vi "Test Lockin Engine.vi"(8 "error in (no error)":errorcluster, 11 "Lockin.DAQ":refnum<class "Instrument.DAQ.lvclass">) -> (0 "error out":errorcluster, 3 "Lockin.DAQ":refnum<class "Instrument.DAQ.lvclass">)   [LabVIEW 2019, in "Instrument.Lockin.lvlib" / "Instrument.DAQ.lvclass"]
uses:
  Instrument.DAQ.lvclass
  DAQmx/DAQmx.lvclass
  <vilib>/Analysis/NI_AALBase.lvlib
  <vilib>/Analysis/baseanly.llb/Mean (DBL).vi
  C:/Program Files/National Instruments/LabVIEW 2019/vi.lib/JKI/JKI SMO/SMO/SMO.lvclass
  Typedefs/AO.Channel.Function--Enum.ctl
  Typedefs/AO.Channel--Cluster--Array.ctl
  Typedefs/DAQ.Sampling.Sampling--Cluster.ctl
  Typedefs/AO.Channel--Cluster.ctl
  Typedefs/REF.Channel--Cluster.ctl
  Typedefs/REF.Channel--Cluster--Array.ctl
  Typedefs/AI.Channel--Cluster.ctl
  Typedefs/AI.Channel--Cluster--Array.ctl
panel:
  in  "Configuration.AI Channels":T1=[{"Enable?"=TRUE, "Channel"=1, "References"=[1], "reference index"=0}] {"reference index" min=1; "References" items=["", "1", "2", "3", "4", "5", "6", "7", "8", "9"]; "Channel" min=1}
  in  "Configuration.Channels: REF":T3=[{"Enable?"=TRUE, "Channel"=1, "Frequency"=13.0, "Phase"=0.0, "TC"=0.1, "Roll-Off"=2}] {"Roll-Off" min=1 max=4; "TC" min=1e-06 max=100.0 format="%#_3p"; "Phase" format="%#_3p"; "Frequency" min=1e-06 max=102400.0 format="%#_6p"; "Channel" min=1}
  out "refresh rate (Hz)":dbl=13.0
  out "Waveform Graph":dbl[][](graph)=[[0.007605197078202029, 0.03790640341016081, 0.068814310341492]]
  in  "buffer size (samples)":i32=100
  in  "intervals":i32=10
  out "Histogram Graph":T5(graph)
  in  "sampling":T6={"Fs"=204789.0, "#s"=15753} {"Fs" format="%#_13g"}
  in  "Type":enum16{"X", "Y", "R", "Theta", "Mean"}(ring)
  in  "stop":bool
  out "Average time (ms)":dbl=2.3333333333333335
  out "Waveform Chart 2":dbl(graph)
  out "Waveform Chart":dbl[][](graph)=[[0.068814310341492]]
  in  "AO Channels":T7=[{"Enable?"=FALSE, "Channel"=1, "Amplitude"=0.1, "Offset"=0.0, "Frequency"=13.0, "Phase"=0.0, "Function"=enum."sine", "Sweeping?"=FALSE, "Limit AC"=FALSE, "Limit DC?"=FALSE, "Duty Cycle"=FALSE}] {"Phase" format="%#_3g"; "Frequency" min=0.0001 max=200000.0 format="%#_6p"; "Offset" format="%#_6p"; "Amplitude" min=0.0 max=10.0 format="%#_6p"}
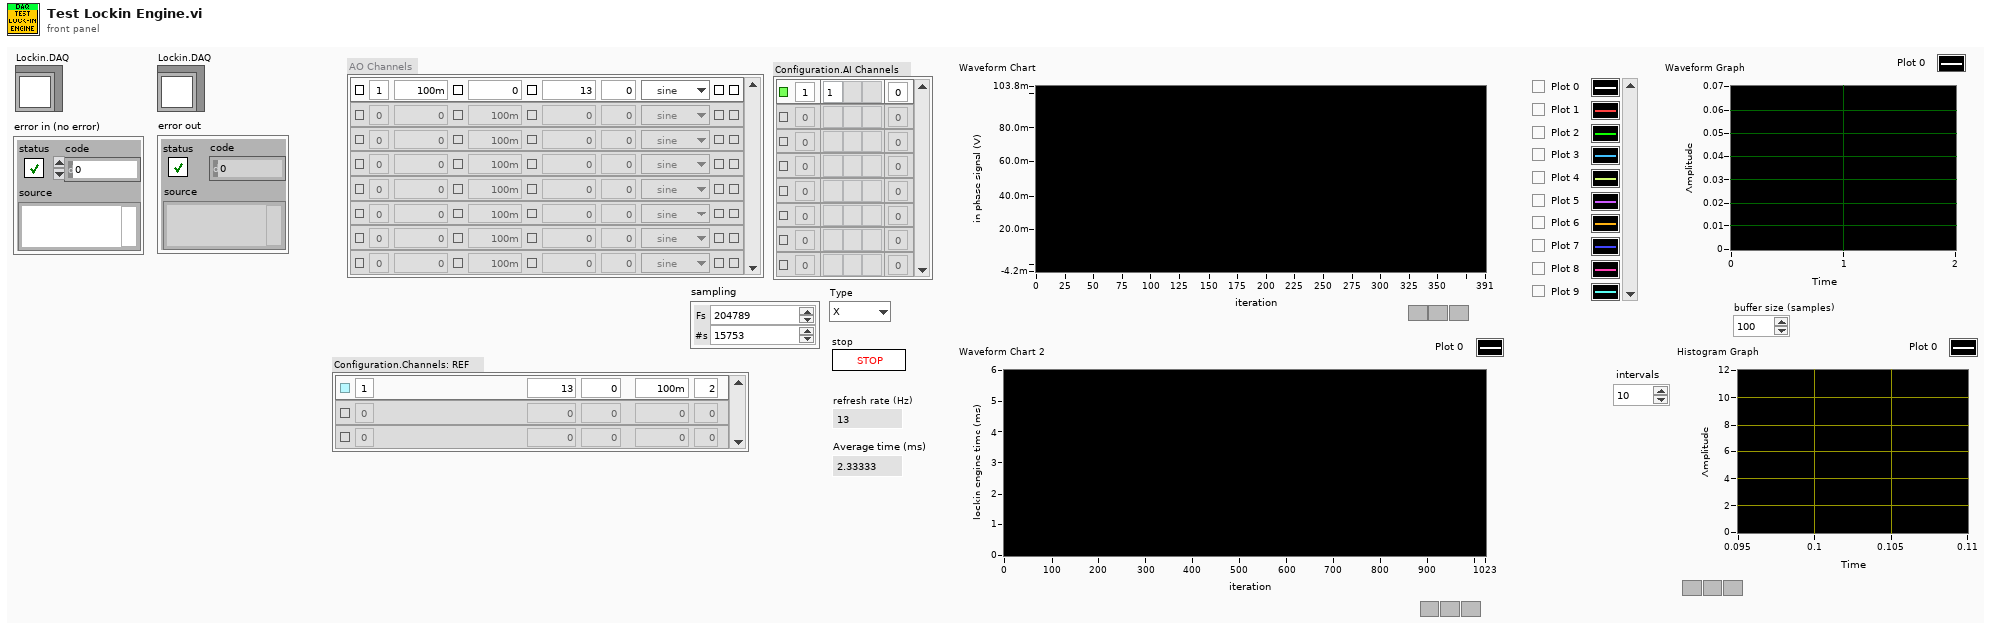
[diagram p1: front panel]
types:
  T1 = typedef "Instrument.Lockin.lvlib/Instrument.DAQ.lvclass/AI.Channel--Cluster--Array.ctl" = T2[]
  T2 = typedef "Instrument.Lockin.lvlib/Instrument.DAQ.lvclass/AI.Channel--Cluster.ctl" = cluster{"Enable?":bool, "Channel":i32, "References":u16[], "reference index":i32}
  T3 = typedef "Instrument.Lockin.lvlib/Instrument.DAQ.lvclass/REF.Channel--Cluster--Array.ctl" = T4[]
  T4 = typedef "Instrument.Lockin.lvlib/Instrument.DAQ.lvclass/REF.Channel--Cluster.ctl" = cluster{"Enable?":bool, "Channel":i32, "Frequency":dbl, "Phase":dbl, "TC":dbl, "Roll-Off":i32}
  T5 = cluster{"X Values":dbl[], "Histogram: h(x)":i32[]}[]
  T6 = typedef "Instrument.Lockin.lvlib/Instrument.DAQ.lvclass/DAQ.Sampling.Sampling--Cluster.ctl" = cluster{"Fs":dbl, "#s":i32}
  T7 = typedef "Instrument.Lockin.lvlib/Instrument.DAQ.lvclass/AO.Channel--Cluster--Array.ctl" = T8[]
  T8 = typedef "Instrument.Lockin.lvlib/Instrument.DAQ.lvclass/AO.Channel--Cluster.ctl" = cluster{"Enable?":bool, "Channel":i32, "Amplitude":dbl, "Offset":dbl, "Frequency":dbl, "Phase":dbl, "Function":T9, "Sweeping?":bool, "Limit AC":bool, "Limit DC?":bool, "Duty Cycle":bool}
  T9 = typedef "Instrument.Lockin.lvlib/Instrument.DAQ.lvclass/AO.Channel.Function--Enum.ctl" = enum16{"sine", "square", "triangle", "saw"}
  T10 = typedef "Instrument.Lockin.lvlib/Instrument.DAQ.lvclass/Results--Cluster.ctl" = cluster{"Time Stamp":timestamp, "Results (Dictionary)":cluster{"key":string, "value":dbl[]}[]}
  T11 = cluster{"X Values":dbl[], "Histogram: h(x)":i32[]}
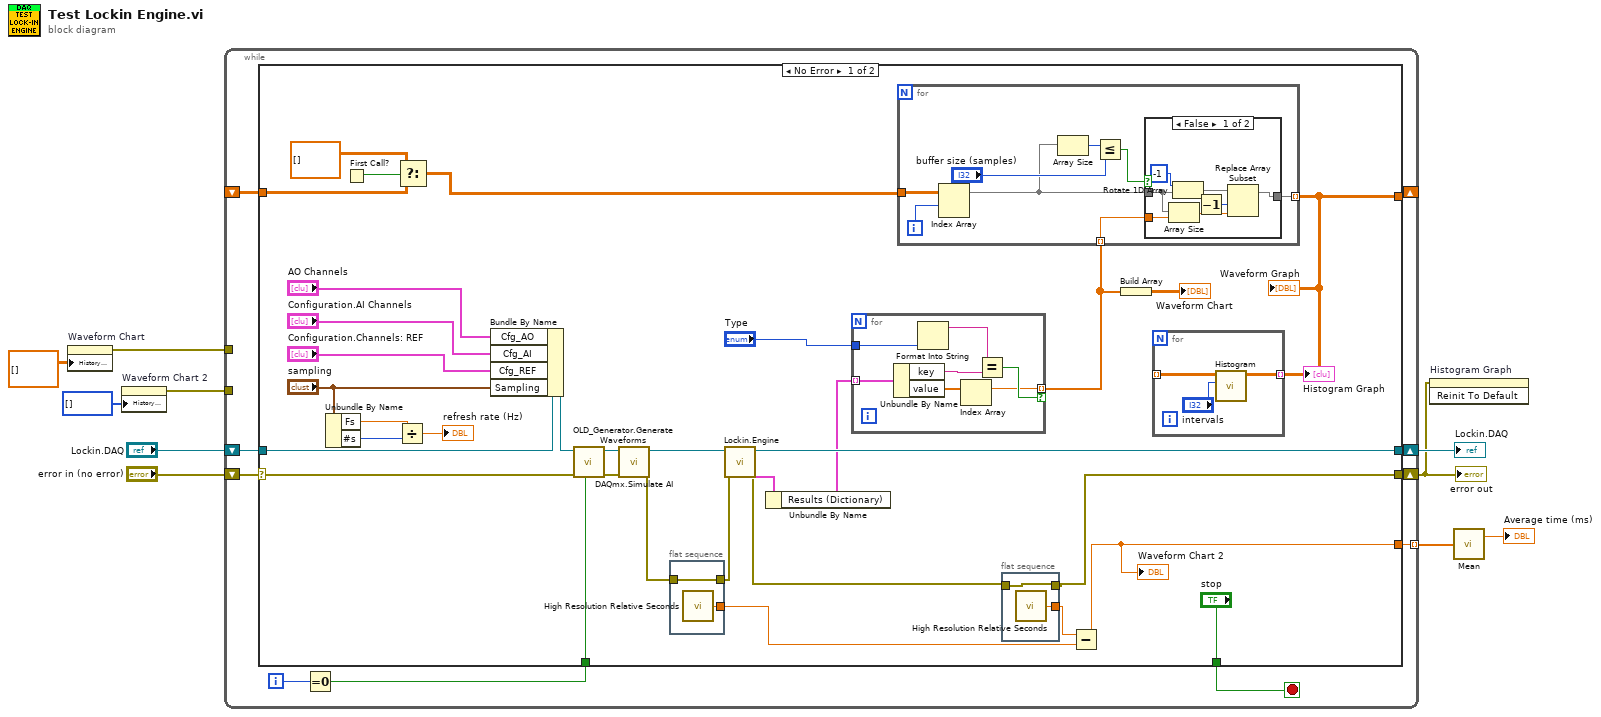
[diagram p0: block diagram]
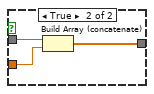
[diagram p2: hidden frame]
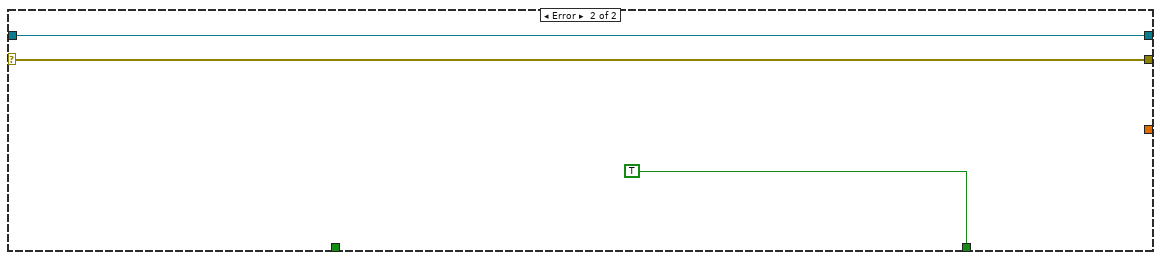
[diagram p3: hidden frame]
diagram:
  n1 = property on="Waveform Chart" class="WFChart (strict)"("History Data"=dbl[][] []) -> (error out=w3:errorcluster)  [unwired: 2 in, 1 out]
  n2 = property on="Waveform Chart 2" class="WFChart (strict)"("History Data"=u32[] []) -> (error out=w4:errorcluster)  [unwired: 2 in, 1 out]
  n3 = while {
    shift-right: [w19] -> w1
    shift-left: "error in (no error)" -> [w20]
    shift-right: [w17] -> w8
    shift-left: "Lockin.DAQ" -> [w18]
    tunnel: [w16] -> w5 mode=indexing
    tunnel: w4 -> [_]
    tunnel: w3 -> [_]
    shift-right: [w12] -> _
    shift-left: _ -> [w11]
    i -> [w14]
    stop <- w13 stop-if-true
    n4 = Equal To 0?(x=w14) -> (x = 0?=w15:bool)
    n5 = case shown="No Error" w20 {
      selector: w20 -> [w53 w89]
      tunnel: [w21 w89] -> w19
      tunnel: [w51 w88] -> w17
      tunnel: w18 -> [w32 w88]
      tunnel: [w48 _] -> w16
      tunnel: w15 -> [w46 _]
      tunnel: ["stop" TRUE ("stop")] -> w13
      tunnel: [w44 _] -> w12
      tunnel: w11 -> [w39 _]
      frame No Error {
        n6 = Unbundle By Name("sampling") -> ("Fs"=w38:dbl, "#s"=w37:i32)
        n7 = First Call?() -> (First Call?: T/F=w41:bool)
        n8 = Divide(x=w38, y=w37) -> (x/y=→"refresh rate (Hz)":dbl)
        n9 = Select(t=dbl[][] [], s=w41, f=w39) -> (s? t:f=w40:dbl[][])
        n10 = Bundle By Name(cluster=w32, "Cfg_AO"="AO Channels", "Cfg_AI"="Configuration.AI Channels", "Cfg_REF"="Configuration.Channels: REF", "Sampling"="sampling") -> (w34:refnum<class "Instrument.DAQ.lvclass">)
        n11 = call "OLD_Generator.Generate Waveforms.vi"("reset phase?"=w46, "error in (no error)"=w53, "Instrument.DAQ"=w34) -> ("error out"=w30:errorcluster, "Instrument.DAQ"=w54:refnum<class "Instrument.DAQ.lvclass">)  [unwired: 6 in, 1 out]
        n12 = call "DAQmx.Simulate AI.vi"("error in (no error)"=w30, "DAQmx in"=w54) -> ("error out"=w23:errorcluster, "DAQmx out"=w52:refnum<class "DAQmx.lvclass">)  [unwired: 6 in, 2 out]
        n13 = flat-sequence {
          tunnel: [w58] -> w28
          tunnel: [w57] -> w24
          tunnel: w23 -> [w57]
          frame #0 {
            n14 = call <vilib>:"High Resolution Relative Seconds.vi"() -> ("relative seconds"=w58:dbl)
          }
        }
        n15 = call "Lockin.Engine.vi"("error in (no error)"=w24, "Instrument.DAQ"=w52) -> ("error out"=w22:errorcluster, "Results (X,Y,R,Theta,Mean)"=w50:T10, "Instrument.DAQ out"=w51:refnum<class "Instrument.DAQ.lvclass">)  [unwired: 5 in, 2 out]
        n16 = Unbundle By Name(w50) -> ("Results (Dictionary)"=w27:cluster{"key":string, "value":dbl[]}[])
        n17 = for {
          tunnel: w27 -> [w65] mode=indexing
          tunnel: "Type" -> [w64]
          tunnel: [w59] -> w25 mode=indexing if=w60
          n18 = Unbundle By Name(w65) -> ("key"=w62:string, "value"=w61:dbl[])
          n19 = Format Into String(w64) -> (resulting string=w63:string)  [unwired: 3 in, 1 out]
          n20 = Index Array(array=w61) -> (element=w59:dbl)  [unwired: 1 in]
          n21 = Equal?(x=w63, y=w62) -> (x = y?=w60:bool)
        }
        n22 = for {
          tunnel: w40 -> [w76]
          tunnel: [w72] -> w44 mode=indexing
          tunnel: w25 -> [w71] mode=indexing
          i -> [w69]
          n23 = Index Array(array=w76, index (row)=w69) -> (element=w70:dbl[])  [unwired: 1 in]
          n24 = Array Size(array=w70) -> (size(s)=w75:i32)
          n25 = Less Or Equal?(x=w75, y="buffer size (samples)") -> (x <= y?=w73:bool)
          n26 = case shown="False" w73 {
            tunnel: [w78 w86] -> w72
            tunnel: w71 -> [w81 w84]
            tunnel: w70 -> [w80 w85]
            frame False {
              n27 = Array Size(array=w80) -> (size(s)=w79:i32)
              n28 = Rotate 1D Array(1:w80, 2:-1 ("n")) -> (0:w82:dbl[])
              n29 = Decrement(x=w79) -> (x-1=w77:i32)
              n30 = Replace Array Subset(array=w82, new element=w81, index=w77) -> (w78:dbl[])
            }
            frame True {
              n31 = Build Array (concatenate)(w85, w84) -> (w86:dbl[])
            }
          }
        }
        "Waveform Graph" <- w44
        n32 = flat-sequence {
          tunnel: [w56] -> w49
          tunnel: [w55] -> w21
          tunnel: w22 -> [w55]
          frame #0 {
            n33 = call <vilib>:"High Resolution Relative Seconds.vi"() -> ("relative seconds"=w56:dbl)
          }
        }
        n34 = Subtract(x=w49, y=w28) -> (x-y=w48:dbl)
        "Waveform Chart 2" <- w48
        n35 = Build Array(w25) -> (→"Waveform Chart":dbl[][])
        n36 = for {
          tunnel: w44 -> [w67] mode=indexing
          tunnel: [w66] -> w43 mode=indexing
          n37 = call <vilib>:"Histogram.vi"("intervals"="intervals", "X"=w67) -> ("Histogram Graph"=w66:T11)  [unwired: 6 in, 3 out]
        }
        "Histogram Graph" <- w43
      }
      frame Error {
      }
    }
  }
  "error out" <- w1
  "Lockin.DAQ" <- w8
  n38 = invoke on="Histogram Graph" class="XYGraph (strict)" method="Reinit To Default"(error in=w1) -> ()  [unwired: 2 in, 3 out]
  n39 = call-poly <vilib>:"Mean.vi"("X"=w5) -> ("mean"=→"Average time (ms)":dbl)  [unwired: 1 out]
